vi "Testing.vi"() -> ()   [LabVIEW 2021]
panel:
  out "Threshold Reached":bool
  in  "Threshold":dbl
  out "Angle Stack":T1
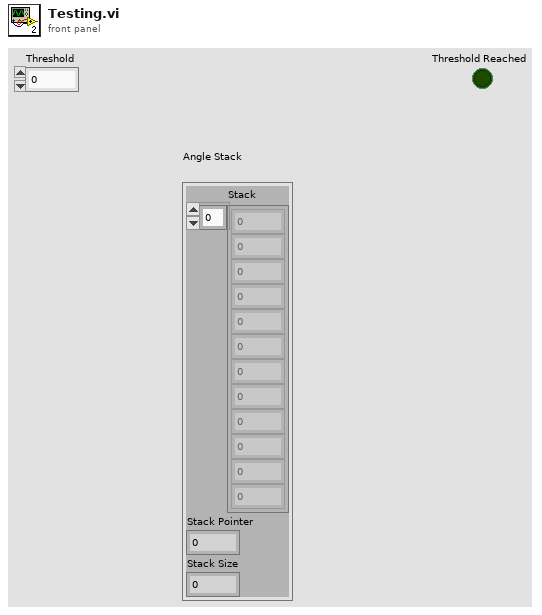
[diagram p1: front panel]
types:
  T1 = cluster{"Stack":dbl[], "Stack Pointer":dbl, "Stack Size":dbl}
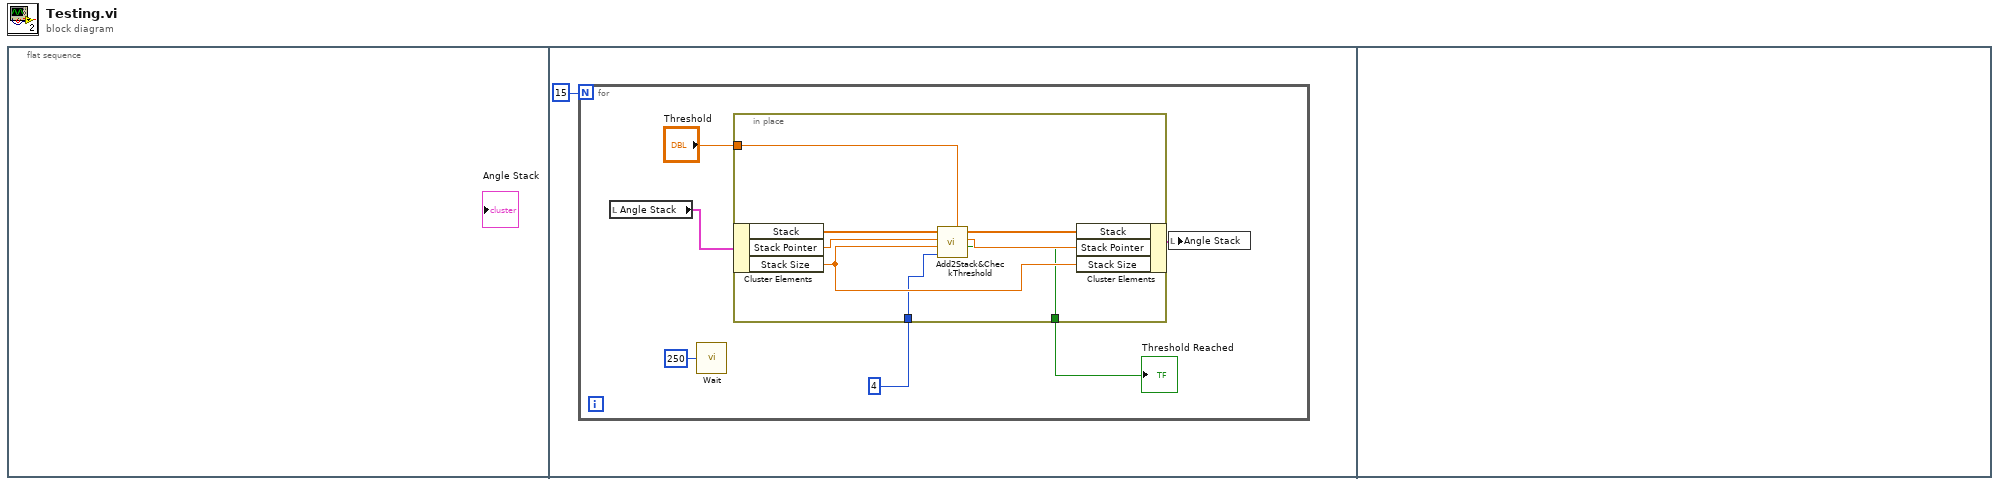
[diagram p0: block diagram]
diagram:
  n1 = flat-sequence {
    frame #0 {
    }
    frame #1 {
      n2 = for {
        N: 15 -> [_]
        n3 = local read "Angle Stack"() -> (w7:T1)
        n4 = call "Wait"("Count(mSec)"=u32 250) -> ()  [unwired: 1 out]
        n5 = in-place {
          in-place-border: 4 -> [w10]
          in-place-border: "Threshold" -> [w9]
          in-place-border: [w8] -> w4
          n6 = in-place-cluster #1(w7) -> ("Stack"=w15:dbl[], "Stack Pointer"=w14:dbl, "Stack Size"=w11:dbl)
          n7 = call "Add2Stack&CheckThreshold.vi"("Stack In"=w15, "Stack Pointer  In"=w14, "Stack Size"=w11, "Angle"=w10, "Threshold"=w9) -> ("Stack Out"=w13:dbl[], "Stack Pointer Out"=w12:dbl, "Threshold Reached"=w8:bool)  [unwired: 2 in]
          n8 = in-place-cluster #1("Stack"=w13, "Stack Pointer"=w12, "Stack Size"=w11) -> (w6:T1)
        }
        "Threshold Reached" <- w4
        n9 = local write "Angle Stack"(w6) -> ()
      }
    }
    frame #2 {
    }
  }
